vi "报警信息.vi"(8 "error in (no error)":errorcluster, 11 "data":T1) -> (0 "error out":errorcluster)   [LabVIEW 2016, in "数据传输系统.lvlib"]
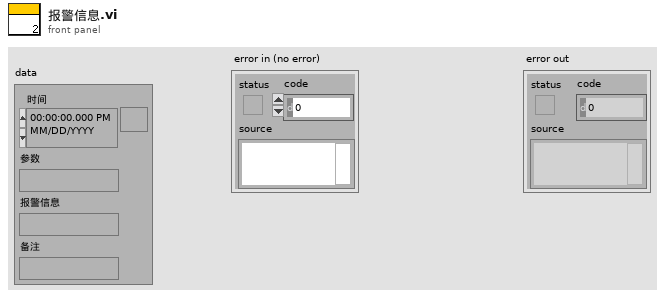
[diagram p1: front panel]
types:
  T1 = typedef "报警信息字段定义.ctl" = cluster{"时间":timestamp, "参数":string, "报警信息":string, "备注":string}
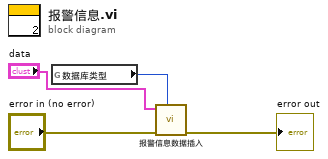
[diagram p0: block diagram]
diagram:
  n1 = global read "断电保存全局.vi" "数据库类型"() -> (w4:enum16{"Access", "SQLite"})
  n2 = call "报警信息数据插入.vi"("data"="data", "错误输入（无错误）"="error in (no error)", "数据库类型"=w4) -> ("错误输出"=→"error out":errorcluster)  [unwired: 7 in]
